vi "PH_ImageOperator.PC Set Beam Analysis.vi"(0 "i ref in":refnum<vi>, 2 "On / Off":bool, 5 "error in":errorcluster) -> (14 "i ref out":refnum<vi>, 19 "error out":errorcluster)   [LabVIEW 2014, in "PH_ImageOperator.lvlib"]
doc: "This VI writes beam analysis settings to own attributes and sets the GUI elements."
uses:
  PH_ImageOperator.lvlib
  CSCore/CSSystem/CSSystemLib/CSSystemLib.lvlib
  PH_Common/PH_Common.lvlib
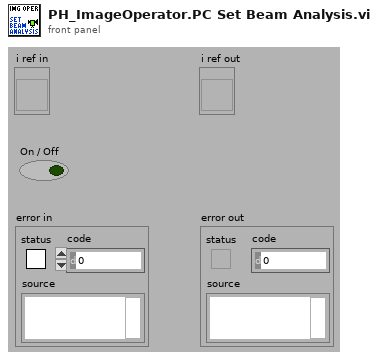
[diagram p1: front panel]
types:
  T1 = typedef "PH_ImageOperator.lvlib/PH_ImageOperator.i attribute.ctl" = cluster{"GUI Refs":cluster{"Delete":refnum<vi>, "Calibration status":refnum<vi>, "BI subtracted":refnum<vi>, "calc Energy":refnum<vi>, "Energy: expected value":refnum<vi>, "Energy: Tolerance":refnum<vi>, "Energy calculated":refnum<vi>, "Energy":refnum<vi>, "calc Beam Anal":refnum<vi>, "Maj Diam 1/esquare":refnum<vi>, "Min Diam 1/esquare":refnum<vi>, "Azi Angle":refnum<vi>, "Min/Maj Diam esquare":refnum<vi>, "Beam analysed":refnum<vi>, "CoG - x":refnum<vi>, "CoG - y":refnum<vi>, "BA: Method":refnum<vi>, "BA: Steps":refnum<vi>, "BA: Factor":refnum<vi>, "calc Traces":refnum<vi>, "Traces: Fit Gauss":refnum<vi>, "Traces calculated":refnum<vi>, "Maj FWHM":refnum<vi>, "Min FWHM":refnum<vi>, "Major Trace":refnum<vi>, "Minor Trace":refnum<vi>, "Maj Fit Order":refnum<vi>, "Min Fit Order":refnum<vi>, "Position calculated":refnum<vi>, "Position":refnum<vi>, "Type":refnum<vi>, "Center":refnum<vi>, "exp - X":refnum<vi>, "exp - Y":refnum<vi>, "Tolerance":refnum<vi>, "f":refnum<vi>, "M":refnum<vi>, "D":refnum<vi>, "q":refnum<vi>, "Dummy Method":refnum<vi>, "Dummy Type":refnum<vi>, "Global On":refnum<vi>, "Traces: No offset":refnum<vi>, "Maj 99%":refnum<vi>, "Min 99%":refnum<vi>, "GUI FF Image":refnum<vi>, "calc Fill Factor":refnum<vi>, "FF calculated":refnum<vi>, "Fill Factor: Filter?":refnum<vi>, "FF: Damage Threshold":refnum<vi>, "FF: Threshold":refnum<vi>, "FF: max allow. Energy":refnum<vi>, "FF: Fillfactor":refnum<vi>, "Calibration data":refnum<vi>}, "List of GUIs":string[], "Calibration":cluster{"Status":T2, "Calibration data":T3, "Calibration Data File":path}, "Final Image":cluster{"BI Subtraction Failure":bool}, "Energy":cluster{"on":bool, "expected value [mJ]":dbl, "Tolerance [%]":dbl, "State":T2, "Energy [mJ]":dbl, "Unit":string, "calculated @":timestamp}, "Beam Analysis":cluster{"on":bool, "Data":T4, "Method":bool, "Steps":i32, "Factor":i32, "ROI":cluster{"Left":i32, "Top":i32, "Right":i32, "Bottom":i32}, "analysed @":timestamp}, "Trace Analysis":cluster{"on":bool, "Fit on":bool, "Maj FWHM":dbl, "Min FWHM":dbl, "Maj Fit Order":i32, "Min Fit Order":i32, "No Offset":bool, "Maj 99%":dbl, "Min 99%":dbl, "Traces":cluster{"XScaleName":string, "Y Scale Minimum":sgl, "Y Scale Maximum":sgl, "X Scale Minimum":sgl, "X Scale Maximum":sgl, "Traces":cluster{"Index":sgl[], "Trace":dbl[]}[]}[], "analysed @":timestamp}, "Position Analysis":cluster{"on":bool, "exp - X":i32, "exp - Y":i32, "focal length [mm]":dbl, "Magnification":dbl, "Delta":dbl, "Theta":dbl, "Tolerance":dbl, "Type":bool, "analysed @":timestamp}, "Fill Factor":cluster{"on":bool, "Filter on?":bool, "Threshold":dbl, "Damage Threshold [J/cm²]":dbl, "Fillfactor":dbl, "Max. allowed Energy [J]":dbl, "calculated @":timestamp}, "Statistician Service ID":i32, "Images":cluster{"Background":T5, "OP":T5, "GUI":T5, "BA: ROI":T5, "Trace: Turn":T5, "FF: Main":T5, "FF: Help":T5, "PSDB: BG":T5, "PSDB: OP":T5, "PSDB: FF":T5}}
  T2 = typedef "PH_StatusHandler.lvlib/PH_StatusHandler.Status.ctl" = i16
  T3 = typedef "PH_ImageCalibrator.lvlib/PH_ImageCalibrator.Calibration Data.ctl" = cluster{"Date":string, "Time":string, "Cam Settings":cluster{"Cam ID":string, "Gain":dbl, "Brightness":dbl, "Shutter":dbl, "Cam Error":bool, "Mode":i32}, "Background Image":cluster{"Image":dbl[][], "Image Error":bool}, "Linear Calibration":cluster{"Calibration Factor":dbl, "not mm or mrad":bool}, "Energy Calibration":cluster{"Calibration Factor":dbl, "no mJ":bool}}
  T4 = typedef "PH_ImageOperator.lvlib/PH_ImageOperator.Beam Analysis Data.ctl" = cluster{"CoG-x":sgl, "CoG-y":sgl, "Maj Dim":dbl, "Min Dim":dbl, "Ellipticity":dbl, "Azimuth Angle [rad]":dbl, "Azi Angle rel to Maj?":bool}
  T5 = typedef "IMAQ Image.ctl" = refnum<image>
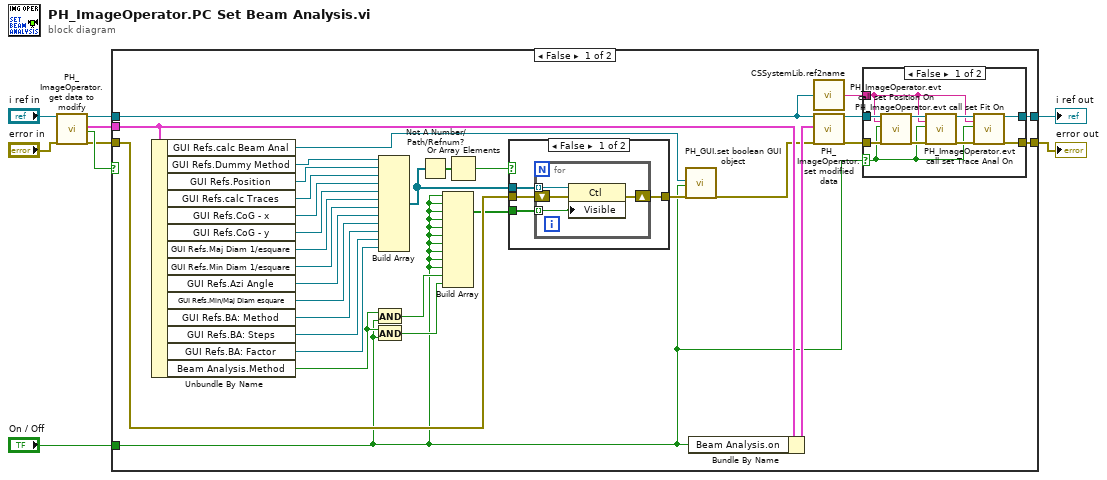
[diagram p0: block diagram]
diagram:
  n1 = call "PH_ImageOperator.get data to modify.vi"("i ref in"="i ref in", "error in (no error)"="error in") -> ("i ref out"=w3:refnum<vi>, "i attribute"=w8:T1, "timed out"=w7:bool, "error out"=w5:errorcluster)  [unwired: 14 in]
  n2 = case shown="False" w7 {
    tunnel: w3 -> [w16 w64]
    tunnel: [w17 w64] -> w4
    tunnel: w5 -> [w30 w63]
    tunnel: [w19 w63] -> w6
    tunnel: w8 -> [w31 _]
    tunnel: "On / Off" -> [w10 _]
    frame False {
      n3 = Unbundle By Name(w31) -> ("GUI Refs.calc Beam Anal"=w13:refnum<vi>, "GUI Refs.Dummy Method"=w14:refnum<vi>, "GUI Refs.Position"=w21:refnum<vi>, "GUI Refs.calc Traces"=w22:refnum<vi>, "GUI Refs.CoG - x"=w33:refnum<vi>, "GUI Refs.CoG - y"=w34:refnum<vi>, "GUI Refs.Maj Diam 1/esquare"=w35:refnum<vi>, "GUI Refs.Min Diam 1/esquare"=w36:refnum<vi>, "GUI Refs.Azi Angle"=w37:refnum<vi>, "GUI Refs.Min/Maj Diam esquare"=w38:refnum<vi>, "GUI Refs.BA: Method"=w29:refnum<vi>, "GUI Refs.BA: Steps"=w28:refnum<vi>, "GUI Refs.BA: Factor"=w27:refnum<vi>, "Beam Analysis.Method"=w23:bool)
      n4 = And(x=w23, y=w10) -> (x .and. y?=w25:bool)
      n5 = And(x=w23, y=w10) -> (x .and. y?=w24:bool)
      n6 = Build Array(w14, w21, w22, w33, w34, w35, w36, w37, w38, w29, w28, w27) -> (w40:refnum<vi>[])
      n7 = Not A Number/Path/Refnum?(number/path/refnum=w40) -> (NaN/Path/Refnum?=w32:bool[])
      n8 = Build Array(w10, w10, w10, w10, w10, w10, w10, w10, w10, w10, w25, w24) -> (w26:bool[])
      n9 = Or Array Elements(Boolean array=w32) -> (logical OR=w39:bool)
      n10 = case shown="False" w39 {
        tunnel: w40 -> [w57 _]
        tunnel: w26 -> [w56 _]
        tunnel: [w55 w62] -> w12
        tunnel: w30 -> [w54 w62]
        frame False {
          n11 = for {
            tunnel: w57 -> [w61] mode=indexing
            tunnel: w56 -> [w60] mode=indexing
            shift-right: [w58] -> w55
            shift-left: w54 -> [w59]
            n12 = property class="Ctl"(reference=w61, error in=w59, "Visible"=w60) -> (error out=w58:errorcluster)  [unwired: 1 out]
          }
        }
        frame True {
        }
      }
      n13 = call "PH_GUI.set boolean GUI object.vi"("Boolean Knob GUI Ref"=w13, "Value"=w10, "error in (no error)"=w12) -> ("error out"=w11:errorcluster)  [unwired: 16 in]
      n14 = Bundle By Name(cluster=w31, "Beam Analysis.on"=w10) -> (w41:T1)
      n15 = call "CSSystemLib.ref2name.vi"("obj refnum"=w16) -> ("name"=w15:string)
      n16 = call "PH_ImageOperator.set modified data.vi"("i ref in"=w16, "i attribute"=w41, "error in (no error)"=w11) -> ("i ref out"=w18:refnum<vi>, "error out"=w20:errorcluster)  [unwired: 15 in]
      n17 = case shown="False" w10 {
        selector: w10 -> [w42 _]
        tunnel: w20 -> [w51 w52]
        tunnel: [w46 w52] -> w19
        tunnel: w18 -> [w50 w53]
        tunnel: [w44 w53] -> w17
        tunnel: w15 -> [w43 _]
        frame False {
          n18 = call "PH_ImageOperator.evt call set Position On.vi"("i ref in"=w50, "Instance"=w43, "Position On"=w42, "error in"=w51) -> ("i ref out"=w48:refnum<vi>, "error out"=w49:errorcluster)  [unwired: 14 in]
          n19 = call "PH_ImageOperator.evt call set Trace Anal On.vi"("i ref in"=w48, "Instance"=w43, "Trace Anal on"=w42, "error in (no error)"=w49) -> ("i ref out"=w45:refnum<vi>, "error out"=w47:errorcluster)  [unwired: 14 in]
          n20 = call "PH_ImageOperator.evt call set Fit On.vi"("i ref in"=w45, "Instance"=w43, "Fit on"=w42, "error in (no error)"=w47) -> ("i ref out"=w44:refnum<vi>, "error out"=w46:errorcluster)  [unwired: 14 in]
        }
        frame True {
        }
      }
    }
    frame True {
    }
  }
  "error out" <- w6
  "i ref out" <- w4
